vi "Config PDC Framed.vi"(0 "VISA Resource Name":refnum<visa-resource-name>, 1 "Frame Trigger (2:TRIGGER KEY)":enum16{"BUS", "EXTERNAL", "TRIGGER KEY"}(ring)=enum."TRIGGER KEY", 2 "Ext Delay (F:OFF)":bool, 3 "Ext Delay Bits (0)":i32, 5 "Frame Repeat (F:CONT)":bool, 7 "Rate (T:FULL)":bool=TRUE, 11 "error in (no error)":errorcluster {"code" format="%.0x"}, 12 "Secondary Frame (F:OFF)":bool, 13 "Sec Frame Trigger (1:EXT)":enum16{"BUS", "EXTERNAL", "TRIGGER KEY"}(ring)=enum."EXTERNAL") -> (4 "VISA Resource Name Out":refnum<visa-resource-name>, 15 "error out":errorcluster {"code" format="%.0x"})   [LabVIEW 2014, in "Agilent ESG Series.lvlib"]
doc: "This VI is used to configure PDC framed data.\nRun the Config PDC framed Timeslot.vi after this vi to configure an individual Timeslot."
uses:
  Agilent ESG Series.lvlib
panel:
  # "SINGLE"
  # "CONT"
  # "FULL"
  # "HALF"
  # "ON"
  # "ON"
  # "OFF"
  # "OFF"
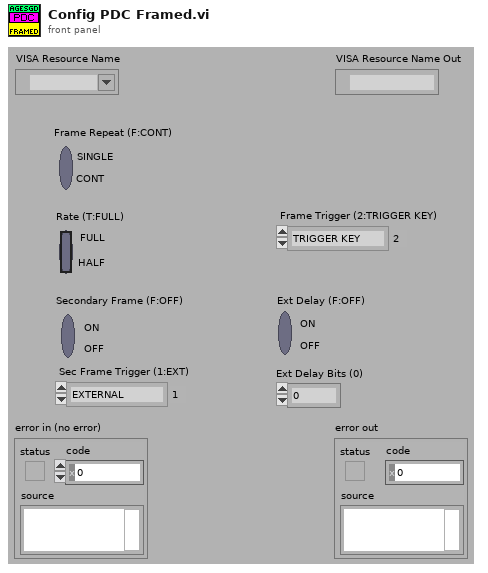
[diagram p1: front panel]
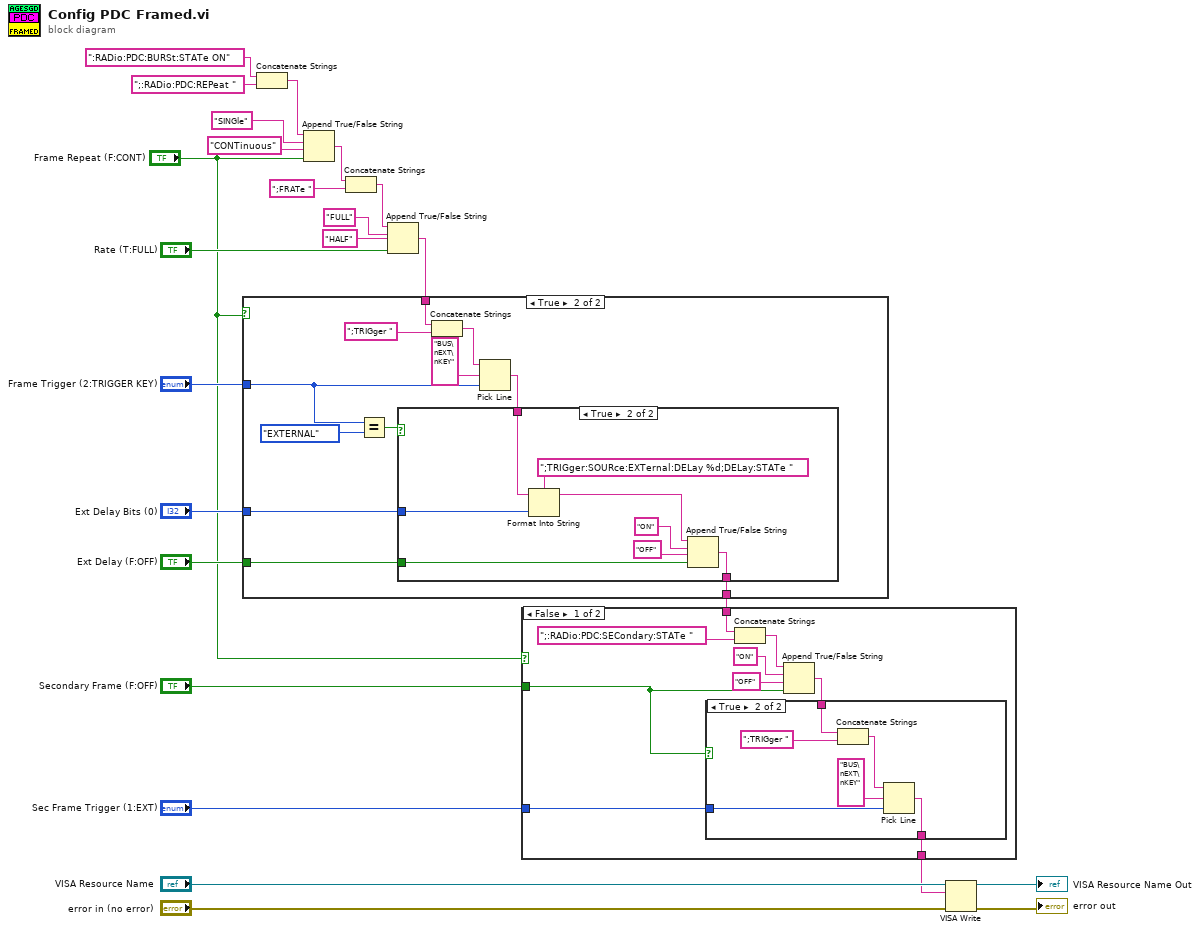
[diagram p0: block diagram]
diagram:
  n1 = Concatenate Strings(":RADio:PDC:BURSt:STATe ON", ";:RADio:PDC:REPeat ") -> (w17:string)
  n2 = Append True/False String(1:"Frame Repeat (F:CONT)", 2:"CONTinuous" ("false string"), 3:"SINGle" ("true string"), 4:w17) -> (0:w16:string)
  n3 = Concatenate Strings(w16, ";FRATe ") -> (w12:string)
  n4 = Append True/False String(1:"Rate (T:FULL)", 2:"HALF" ("false string"), 3:"FULL" ("true string"), 4:w12) -> (0:w7:string)
  n5 = case shown="True" "Frame Repeat (F:CONT)" {
    tunnel: w7 -> [w25 w34]
    tunnel: [w25 w29] -> w6
    tunnel: "Frame Trigger (2:TRIGGER KEY)" -> [_ w26]
    tunnel: "Ext Delay Bits (0)" -> [_ w28]
    tunnel: "Ext Delay (F:OFF)" -> [_ w27]
    frame False {
    }
    frame True {
      n6 = Equal?(x=w26, y=enum16{"BUS", "EXTERNAL", "TRIGGER KEY"}."EXTERNAL") -> (x = y?=w30:bool)
      n7 = Concatenate Strings(w34, ";TRIGger ") -> (w33:string)
      n8 = Pick Line(string ("")=w33, multi-line string="BUS\nEXT\nKEY", line index=w26) -> (output string=w32:string)
      n9 = case shown="True" w30 {
        tunnel: w32 -> [w37 w42]
        tunnel: [w37 w40] -> w29
        tunnel: w28 -> [_ w39]
        tunnel: w27 -> [_ w38]
        frame False {
        }
        frame True {
          n10 = Format Into String(format string=";TRIGger:SOURce:EXTernal:DELay %d;DELay:STATe ", initial string=w42, w39) -> (resulting string=w41:string)  [unwired: 1 in, 1 out]
          n11 = Append True/False String(1:w38, 2:"OFF" ("false string"), 3:"ON" ("true string"), 4:w41) -> (0:w40:string)
        }
      }
    }
  }
  n12 = case shown="False" "Frame Repeat (F:CONT)" {
    tunnel: [w54 w62] -> w3
    tunnel: "Secondary Frame (F:OFF)" -> [w53 _]
    tunnel: "Sec Frame Trigger (1:EXT)" -> [w52 _]
    tunnel: w6 -> [w51 w62]
    frame False {
      n13 = Concatenate Strings(w51, ";:RADio:PDC:SECondary:STATe ") -> (w48:string)
      n14 = Append True/False String(1:w53, 2:"OFF" ("false string"), 3:"ON" ("true string"), 4:w48) -> (0:w49:string)
      n15 = case shown="True" w53 {
        tunnel: w49 -> [w55 w58]
        tunnel: [w55 w57] -> w54
        tunnel: w52 -> [_ w56]
        frame False {
        }
        frame True {
          n16 = Concatenate Strings(w58, ";TRIGger ") -> (w61:string)
          n17 = Pick Line(string ("")=w61, multi-line string="BUS\nEXT\nKEY", line index=w56) -> (output string=w57:string)
        }
      }
    }
    frame True {
    }
  }
  n18 = VISA Write(VISA resource name="VISA Resource Name", write buffer=w3, error in (no error)="error in (no error)") -> (VISA resource name out=→"VISA Resource Name Out":refnum<visa-resource-name>, error out=→"error out":errorcluster)  [unwired: 1 out]
